vi "Build_Read Holding Registers.vi"(8 "error in (no error)":errorcluster, 9 "quantity":u16, 10 "starting address":u16) -> (0 "error out":errorcluster, 3 "MB_PDU":T1={"Function Code"=1, "Data"=[], "RTU_DataBytes"=0})   [LabVIEW 2016, in "MB Master.lvlib"]
doc: "Builds PDU for Read Holding Registers (function code 3)."
uses:
  MB Master.lvlib
  MB_PDU_Cluster.ctl
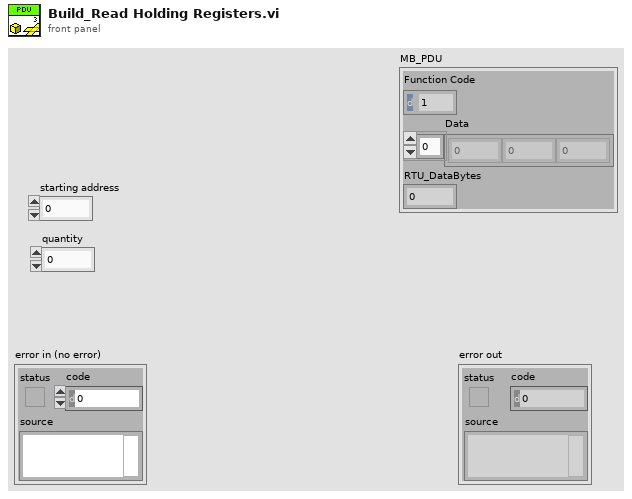
[diagram p1: front panel]
types:
  T1 = typedef "MB Master.lvlib/MB_PDU_Cluster.ctl" = cluster{"Function Code":u8, "Data":u8[], "RTU_DataBytes":i32}
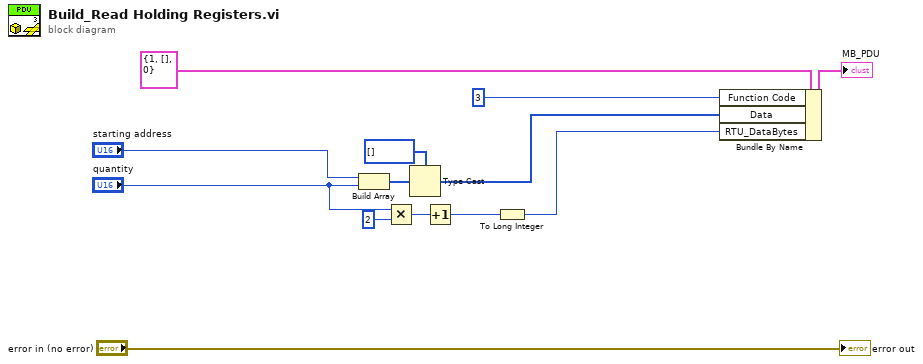
[diagram p0: block diagram]
diagram:
  n1 = Build Array("starting address", "quantity") -> (w13:u16[])
  n2 = Multiply(x="quantity", y=u16 2) -> (x*y=w3:u16)
  n3 = Type Cast(type=u8[] [], x=w13) -> (*(type *) &x=w8:u8[])
  n4 = Increment(x=w3) -> (x+1=w2:u16)
  n5 = To Long Integer(number=w2) -> (32bit integer=w1:i32)
  n6 = Bundle By Name(cluster=T1 {"Function Code"=1, "Data"=[], "RTU_DataBytes"=0} ("Modbus Serial New.lvlib:MB_PDU.lvclass"), "Function Code"=u8 3, "Data"=w8, "RTU_DataBytes"=w1) -> (→"MB_PDU":T1)
  "error out" <- "error in (no error)"
